vi "oax_Get Speed Profile Subset.vi"(8 "error in (no error)":errorcluster, 9 "Duration":dbl=1.0 format="%0.2f", 10 "Start":dbl format="%0.2f", 11 "speed profile":T1 {"speed [RPM]" format="%.2f"; "time [s]" format="%.2f"}) -> (0 "error out":errorcluster, 3 "speed profile out":T1 {"speed [RPM]" format="%.2f"; "time [s]" format="%.2f"})   [LabVIEW 2017]
uses:
  <vilib>/addons/Sound and Vibration/Order Analysis/Tach Process/SubVIs/speed profile.ctl
  <vilib>/addons/Sound and Vibration/Order Analysis/Tach Process/SoundVib_TachProcess.lvlib
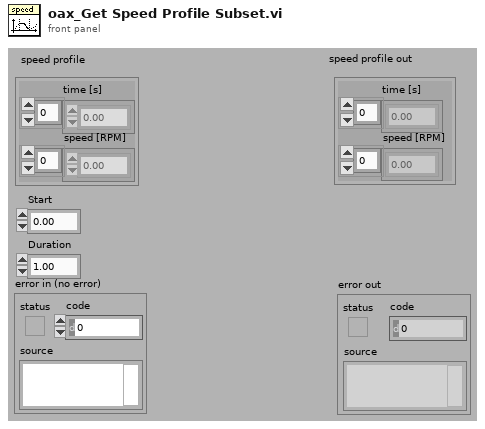
[diagram p1: front panel]
types:
  T1 = typedef "SoundVib_TachProcess.lvlib/speed profile.ctl" = cluster{"time [s]":dbl[], "speed [RPM]":dbl[]}
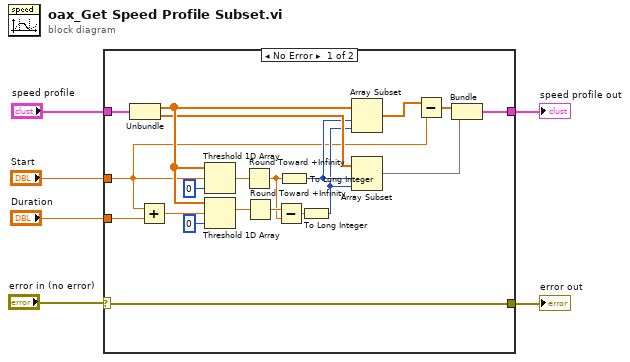
[diagram p0: block diagram]
diagram:
  n1 = case shown="No Error" "error in (no error)" {
    selector: "error in (no error)" -> [w10 w27]
    tunnel: "speed profile" -> [w26 w28]
    tunnel: "Start" -> [w8 _]
    tunnel: "Duration" -> [w22 _]
    tunnel: [w11 w28] -> w2
    tunnel: [w10 w27] -> w1
    frame No Error {
      n2 = Unbundle(w26) -> ("time [s]"=w18:dbl[], "speed [RPM]"=w15:dbl[])
      n3 = Add(x=w8, y=w22) -> (x+y=w21:dbl)
      n4 = Threshold 1D Array(1:0 ("start index (0)"), 2:w8, 3:w18) -> (0:w24:dbl)
      n5 = Threshold 1D Array(1:0 ("start index (0)"), 2:w21, 3:w18) -> (0:w20:dbl)
      n6 = Round Toward +Infinity(x=w24) -> (ceil(x): smallest int >= x=w17:dbl)
      n7 = Round Toward +Infinity(x=w20) -> (ceil(x): smallest int >= x=w19:dbl)
      n8 = Subtract(x=w19, y=w17) -> (x-y=w16:dbl)
      n9 = To Long Integer(number=w17) -> (32bit integer=w14:i32)
      n10 = To Long Integer(number=w16) -> (32bit integer=w13:i32)
      n11 = Array Subset(array=w18, index=w14, length=w13) -> (w9:dbl[])
      n12 = Array Subset(array=w15, index=w14, length=w13) -> (w12:dbl[])
      n13 = Subtract(x=w9, y=w8) -> (x-y=w7:dbl[])
      n14 = Bundle(w7, w12) -> (w11:cluster{dbl[], dbl[]})  [unwired: 1 in]
    }
    frame Error {
    }
  }
  "speed profile out" <- w2
  "error out" <- w1
